vi "setParameters.vi"(10 "Parameters":T1, 11 "EnterMaintenanceCommand in":refnum<class "EnterMaintenanceCommand.lvclass">) -> (3 "EnterMaintenanceCommand out":refnum<class "EnterMaintenanceCommand.lvclass">)   [LabVIEW 2016, in "EnterMaintenanceCommand.lvclass"]
uses:
  EnterMaintenanceCommand.lvclass
  DataTypes/Topics/CommandEnterMaintenance.ctl
  DataTypes/Topics/Parts/CommandId.ctl
  EnterMaintenanceCommand.lvclass/EnterMaintenanceCommand.ctl
  DataTypes/Topics/M1M3SupportTopics.lvlib
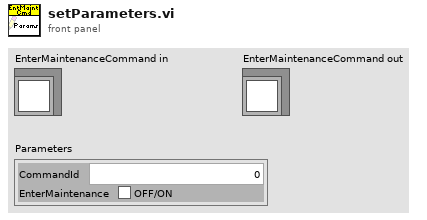
[diagram p1: front panel]
types:
  T1 = typedef "M1M3SupportTopics.lvlib/CommandEnterMaintenance.ctl" = cluster{"CommandId":T2, "EnterMaintenance":bool}
  T2 = typedef "M1M3SupportTopics.lvlib/CommandId.ctl" = i32
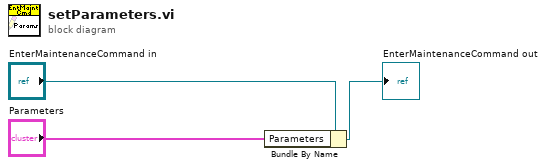
[diagram p0: block diagram]
diagram:
  n1 = Bundle By Name(cluster="EnterMaintenanceCommand in", "Parameters"="Parameters") -> (→"EnterMaintenanceCommand out":refnum<class "EnterMaintenanceCommand.lvclass">)
